vi "niScope Initialize.vi"(0 "resource name":refnum<k15>="DAQ::1", 5 "id query":bool, 9 "reset device":bool=TRUE, 11 "error in":errorcluster) -> (4 "instrument handle":refnum<k15>, 15 "error out":errorcluster)   [LabVIEW 2013]
doc: "Performs the following initialization actions:\n\n--Creates a new IVI instrument driver session.\n\n-Opens a session to the device that you specify in the resource name parameter.\n\n-Queries the instrument ID and checks that it is valid for this instrument driver, if the id query parameter is set to TRUE.\n\n-Resets the instrument to a known state if the reset device parameter is set to TRUE; refer to niScope Reset for the default state of each digitizer.\n\n-Sends initialization commands to set the instrument to the state necessary for the operation of the instrument driver.\n\n-Returns an instrument handle that you use to identify the instrument in all subsequent instrument driver VI calls."
uses:
  niScope_32.dll
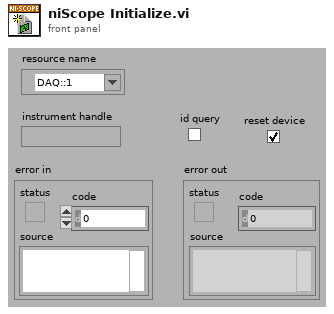
[diagram p1: front panel]
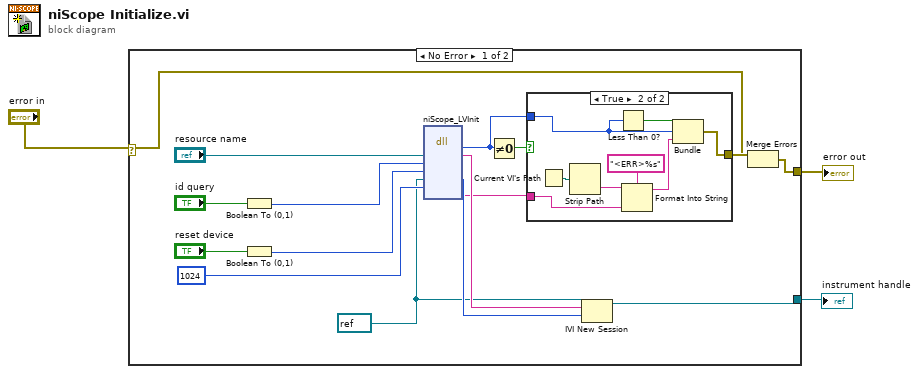
[diagram p0: block diagram]
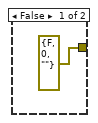
[diagram p2: hidden frame]
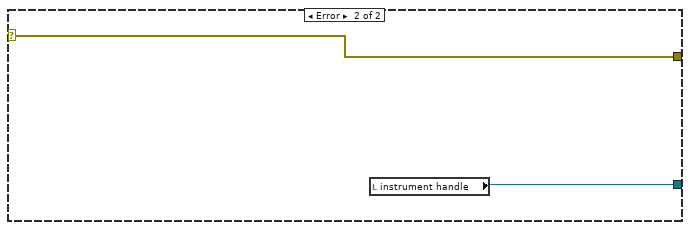
[diagram p3: hidden frame]
diagram:
  n1 = case shown="No Error" "error in" {
    selector: "error in" -> [w5 w29]
    tunnel: [w6 w29] -> w3
    tunnel: [w14 w30] -> w2
    frame No Error {
      w4 = refnum<k15> refnum
      n2 = Boolean To (0,1)(Boolean="id query") -> (0, 1=w16:i16)
      n3 = Boolean To (0,1)(Boolean="reset device") -> (0, 1=w15:i16)
      n4 = dll-call lib="niScope_*.*" fn="niScope_LVInit"("resourceName"="resource name", "IDQuery"=w16, "resetDevice"=w15, "instrument handle"=w4, "error buffer size"=1024) -> ("status"=w10:i32, "resourceName"=w13:string, "instrument handle"=w12:u32, "error buffer"=w8:string)  [unwired: 7 in, 2 out]
      n5 = Not Equal To 0?(x=w10) -> (x != 0?=w11:bool)
      n6 = case shown="True" w11 {
        tunnel: w8 -> [_ w28]
        tunnel: w10 -> [_ w23]
        tunnel: [cluster{bool, "status":i32, string} {FALSE, "status"=0, ""} w21] -> w7
        frame False {
        }
        frame True {
          n7 = Current VI's Path() -> (path=w26:path)
          n8 = Strip Path(path=w26) -> (name=w25:string)  [unwired: 1 out]
          n9 = Less Than 0?(x=w23) -> (x < 0?=w22:bool)
          n10 = Format Into String(format string="<ERR>%s", initial string=w25, w28) -> (resulting string=w24:string)  [unwired: 1 in, 1 out]
          n11 = Bundle(w22, "status"=w23, w24) -> (w21:cluster{bool, "status":i32, string})  [unwired: 1 in]
        }
      }
      n12 = IVI New Session(9:w12, 10:w13, 11:w4) -> (3:w14:refnum<k15>)
      n13 = Merge Errors(w5, w7) -> (w6:errorcluster)
    }
    frame Error {
      n14 = local read "instrument handle"() -> (w30:refnum<k15>)
    }
  }
  "error out" <- w3
  "instrument handle" <- w2
